vi "PPS_TRAJ_BEGIN.vi"(9 "Initial Gyo Reading":T3 {"SIN" format="%13.4f"; "COS" format="%13.4f"; "VALUE" format="%13.4f"}, 10 "Robot Starting Pose":T1 {"ROTATION"."SIN" format="%13.4f"; "ROTATION"."COS" format="%13.4f"; "ROTATION"."VALUE" format="%13.4f"; "TRANSLATION"."Y" format="%14.3f"; "TRANSLATION"."X" format="%14.3f"}, 11 "SWERVE_DRIVE_KINEMATICS":T4 {"SavedModuleStates"."Angle"."SIN" format="%13.4f"; "SavedModuleStates"."Angle"."COS" format="%13.4f"; "SavedModuleStates"."Angle"."VALUE" format="%13.4f"; "PrevCoR"."Y" format="%14.3f"; "PrevCoR"."X" format="%14.3f"; "Modules"."Y" format="%14.3f"; "Modules"."X" format="%14.3f"}) -> ()   [LabVIEW 2019]
uses:
  <vilib>/Rock Robotics/WPI/ThirdParty/JAS_Junk/TrajLib/TypeDef/SWERVE_DRIVE_KINEMATICS.ctl
  <vilib>/Analysis/Matrix/Datatypes/RealMatrix.ctl
  <vilib>/Rock Robotics/WPI/ThirdParty/JAS_Junk/TrajLib/TypeDef/TRANSLATION2D.ctl
  <vilib>/Rock Robotics/WPI/ThirdParty/JAS_Junk/TrajLib/TypeDef/SWERVE_DRIVE_MODULE_STATE.ctl
  <vilib>/Rock Robotics/WPI/ThirdParty/JAS_Junk/TrajLib/TypeDef/ROTATION2D.ctl
  <vilib>/Rock Robotics/WPI/ThirdParty/JAS_Junk/TrajLib/TypeDef/POSE2D.ctl
  PPS_TRAJECTORY_GLOBALS.vi
  <vilib>/Analysis/Matrix/NI_Matrix.lvlib
  <vilib>/Rock Robotics/WPI/ThirdParty/JAS_Junk/TrajLib/Trajectory_Library.lvlib
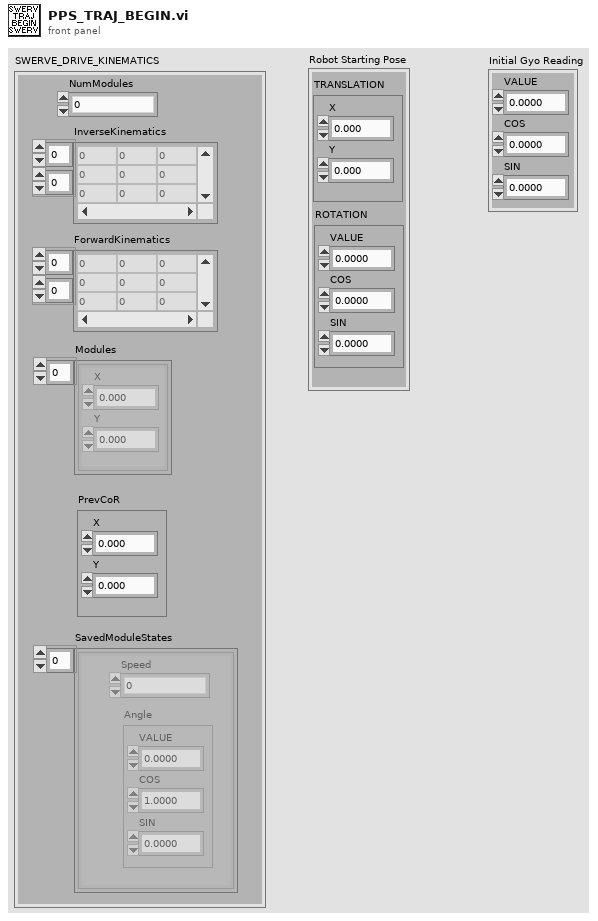
[diagram p1: front panel]
types:
  T1 = typedef "Trajectory_Library.lvlib/POSE2D.ctl" = cluster{"TRANSLATION":T2, "ROTATION":T3}
  T2 = typedef "Trajectory_Library.lvlib/TRANSLATION2D.ctl" = cluster{"X":dbl, "Y":dbl}
  T3 = typedef "Trajectory_Library.lvlib/ROTATION2D.ctl" = cluster{"VALUE":dbl, "COS":dbl, "SIN":dbl}
  T4 = typedef "Trajectory_Library.lvlib/SWERVE_DRIVE_KINEMATICS.ctl" = cluster{"NumModules":i32, "InverseKinematics":T5, "ForwardKinematics":T5, "Modules":T2[], "PrevCoR":T2, "SavedModuleStates":T6[]}
  T5 = typedef "NI_Matrix.lvlib/RealMatrix.ctl" = dbl[][]
  T6 = typedef "Trajectory_Library.lvlib/SWERVE_DRIVE_MODULE_STATE.ctl" = cluster{"Speed":dbl, "Angle":T3}
  T7 = typedef "Trajectory_Library.lvlib/TRAJECTORY.ctl" = cluster{"TotalTImeSecs":dbl, "States":T8[]}
  T8 = typedef "Trajectory_Library.lvlib/TRAJ_STATE.ctl" = cluster{"TimeSeconds":dbl, "Velocity":dbl, "Acceleration":dbl, "POSE":T1, "Curvature":dbl}
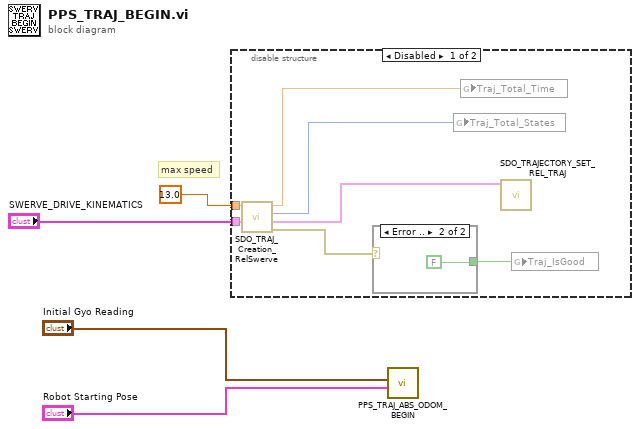
[diagram p0: block diagram]
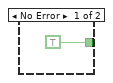
[diagram p2: hidden frame]
diagram:
  # "max speed"
  n1 = disable-structure shown="Disabled" {
    disable-tunnel: 13.0 ("Max Velocity Ft/Sec") -> [w7 _]
    disable-tunnel: "SWERVE_DRIVE_KINEMATICS" -> [w6 _]
    frame Disabled {
      n2 = call "SDO_TRAJ_Creation_RelSwerve.vi"("SWERVE_DRIVE_KINEMATICS"=w6, "Max Velocity Ft/Sec"=w7) -> ("Trajectory  creation error"=w10:errorcluster, "Relative Trajectory"=w5:T7, "Trajectory Items"=w8:i32, "TotalTImeSecs"=w9:dbl)  [unwired: 6 in]
      n3 = case shown="Error .." w10 {
        tunnel: [TRUE FALSE] -> w11
        frame No Error {
        }
        frame Error {
        }
      }
      n4 = global write "PPS_TRAJECTORY_GLOBALS.vi" "Traj_Total_States"(w8) -> ()
      n5 = global write "PPS_TRAJECTORY_GLOBALS.vi" "Traj_Total_Time"(w9) -> ()
      n6 = call "SDO_TRAJECTORY_SET_REL_TRAJ.vi"("Relative_Trajectory"=w5) -> ()  [unwired: 11 in]
      n7 = global write "PPS_TRAJECTORY_GLOBALS.vi" "Traj_IsGood"(w11) -> ()
    }
    frame Enabled {
    }
  }
  n8 = call "PPS_TRAJ_ABS_ODOM_BEGIN.vi"("Initial Pose"="Robot Starting Pose", "Initial Gyro Angle"="Initial Gyo Reading") -> ()  [unwired: 9 in, 1 out]
